vi "Elevator Status.vi"(7 "Action":T1, 8 "error in":errorcluster, 10 "Input":dbl format="%#_13g", 11 "Moving? (F)":bool) -> (0 "error out":errorcluster, 2 "Elevator SP":dbl, 3 "Moving?":bool)   [LabVIEW 2014, in "Elevator System.lvlib"]
uses:
  Elevator System.lvlib
  Typedef/FGVAction.ctl
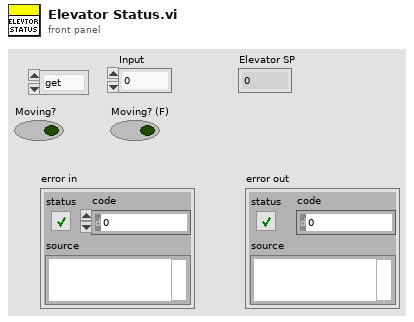
[diagram p1: front panel]
types:
  T1 = typedef "Elevator System.lvlib/FGVAction.ctl" = enum16{"get", "set"}
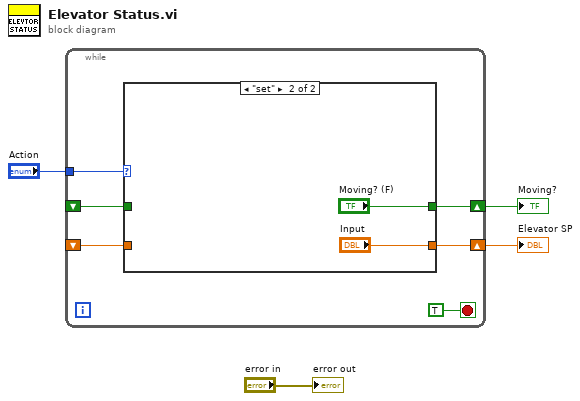
[diagram p0: block diagram]
diagram:
  n1 = while {
    tunnel: "Action" -> [w10]
    shift-right: [w9] -> w2
    shift-left: _ -> [w8]
    shift-right: [w6] -> w1
    shift-left: _ -> [w5]
    stop <- TRUE stop-if-true
    n2 = case shown="\"set\"" w10 {
      tunnel: [w12 "Moving? (F)"] -> w9
      tunnel: w8 -> [w12 _]
      tunnel: [w11 "Input"] -> w6
      tunnel: w5 -> [w11 _]
      frame "get", Default {
      }
      frame "set" {
      }
    }
  }
  "Moving?" <- w2
  "Elevator SP" <- w1
  "error out" <- "error in"
